vi "Read ReadingRate (ms).vi"(8 "error in (no error)":errorcluster, 11 "ElectrometerInternalConfiguration in":refnum<class "ElectrometerInternalConfiguration.lvclass">) -> (0 "error out":errorcluster, 2 "ReadingRate (ms)":dbl, 3 "ElectrometerInternalConfiguration out":refnum<class "ElectrometerInternalConfiguration.lvclass">)   [LabVIEW 2016, in "ElectrometerInternalConfiguration.lvclass"]
uses:
  ElectrometerInternalConfiguration.lvclass
  ElectrometerInternalConfiguration.lvclass/ElectrometerInternalConfiguration.ctl
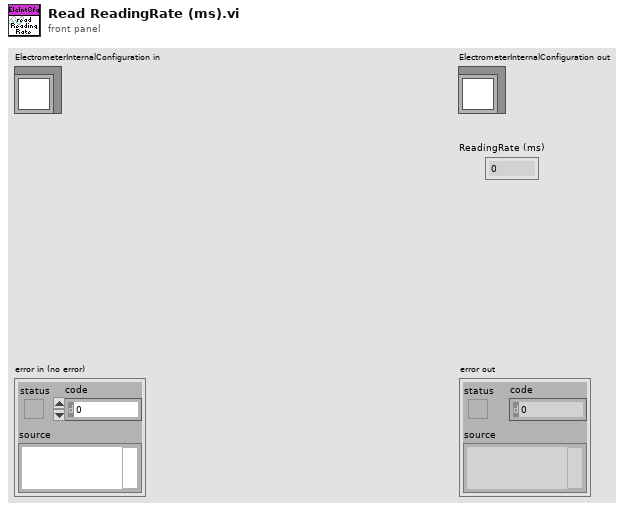
[diagram p1: front panel]
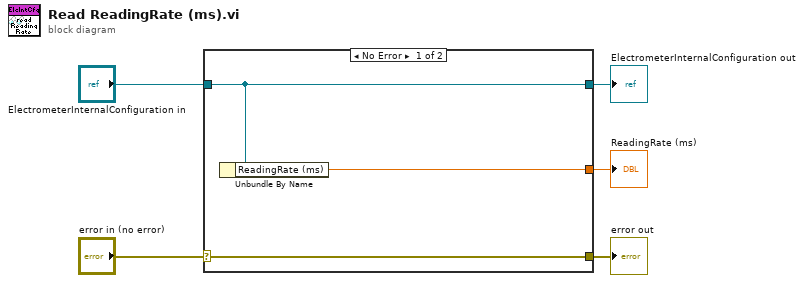
[diagram p0: block diagram]
diagram:
  n1 = case shown="No Error" "error in (no error)" {
    selector: "error in (no error)" -> [w8 w9]
    tunnel: [w8 w9] -> w4
    tunnel: [w7 w10] -> w2
    tunnel: "ElectrometerInternalConfiguration in" -> [w7 w10]
    tunnel: [w6 _] -> w1
    frame No Error {
      n2 = Unbundle By Name(w7) -> ("ReadingRate (ms)"=w6:dbl)
    }
    frame Error {
    }
  }
  "error out" <- w4
  "ElectrometerInternalConfiguration out" <- w2
  "ReadingRate (ms)" <- w1
